vi "Find Circle.vi"(6 "Find Circle Setting":T4={"Options"={"Search  Direction"=0, "Edge Options"={"Edge Polarity"=0, "Kernel Size"=3, "Width"=3, "Minimum Edge Strength"=10.0, "Interpolation Type"=enum."Bilinear Fixed", "Data Processing Method"=enum."Average"}, "Show Search Area"=FALSE, "Show Search Lines"=FALSE, "Show Edges Found"=FALSE, "Show Result"=TRUE, "Search Area Color"=65280, "Search Lines Color"=255, "Edge Locations Color"=16776960, "Result Color"=16711680, "Overlay Group Name"=""}, "Circle Fit Options"={"Process"=enum."Get First Edge", "Step Size"=3.0, "Max Pixel Radius"=3}} {"Options"."Search  Direction" items=["Outside to Inside", "Inside to Outside"]; "Options"."Edge Options"."Edge Polarity" items=["All Edges", "Rising Edges", "Falling Edges"]; "Options"."Edge Options"."Minimum Edge Strength" format="%.2f"; "Options"."Edge Options"."Width" step=2; "Options"."Edge Options"."Kernel Size" step=2}, 8 "error in (no error)":errorcluster, 9 "Matches (pixel)":T7, 10 "ROI Descriptor":T5 {"Contours"."Type" items=["No Selection", "Point", "Line", "Rectangle", "Oval", "Polygon", "Freehand Region", "Annulus", "Unused2", "Unused3", "Broken Line", "Freehand Line", "Rotated Rectangle"]}, 11 "Image":T6) -> (0 "error out":errorcluster, 1 "Fitted Circle":T1, 2 "Found Circle?":bool, 3 "Image Out":T6)   [LabVIEW 2017]
uses:
  <vilib>/vision/Image Controls.llb/IMAQ Image.ctl
  <vilib>/vision/Measure.llb/Edge Options.ctl
  <vilib>/vision/Measure.llb/Edge Polarity.ctl
  <vilib>/vision/NI_Vision_Development_Module.lvlib
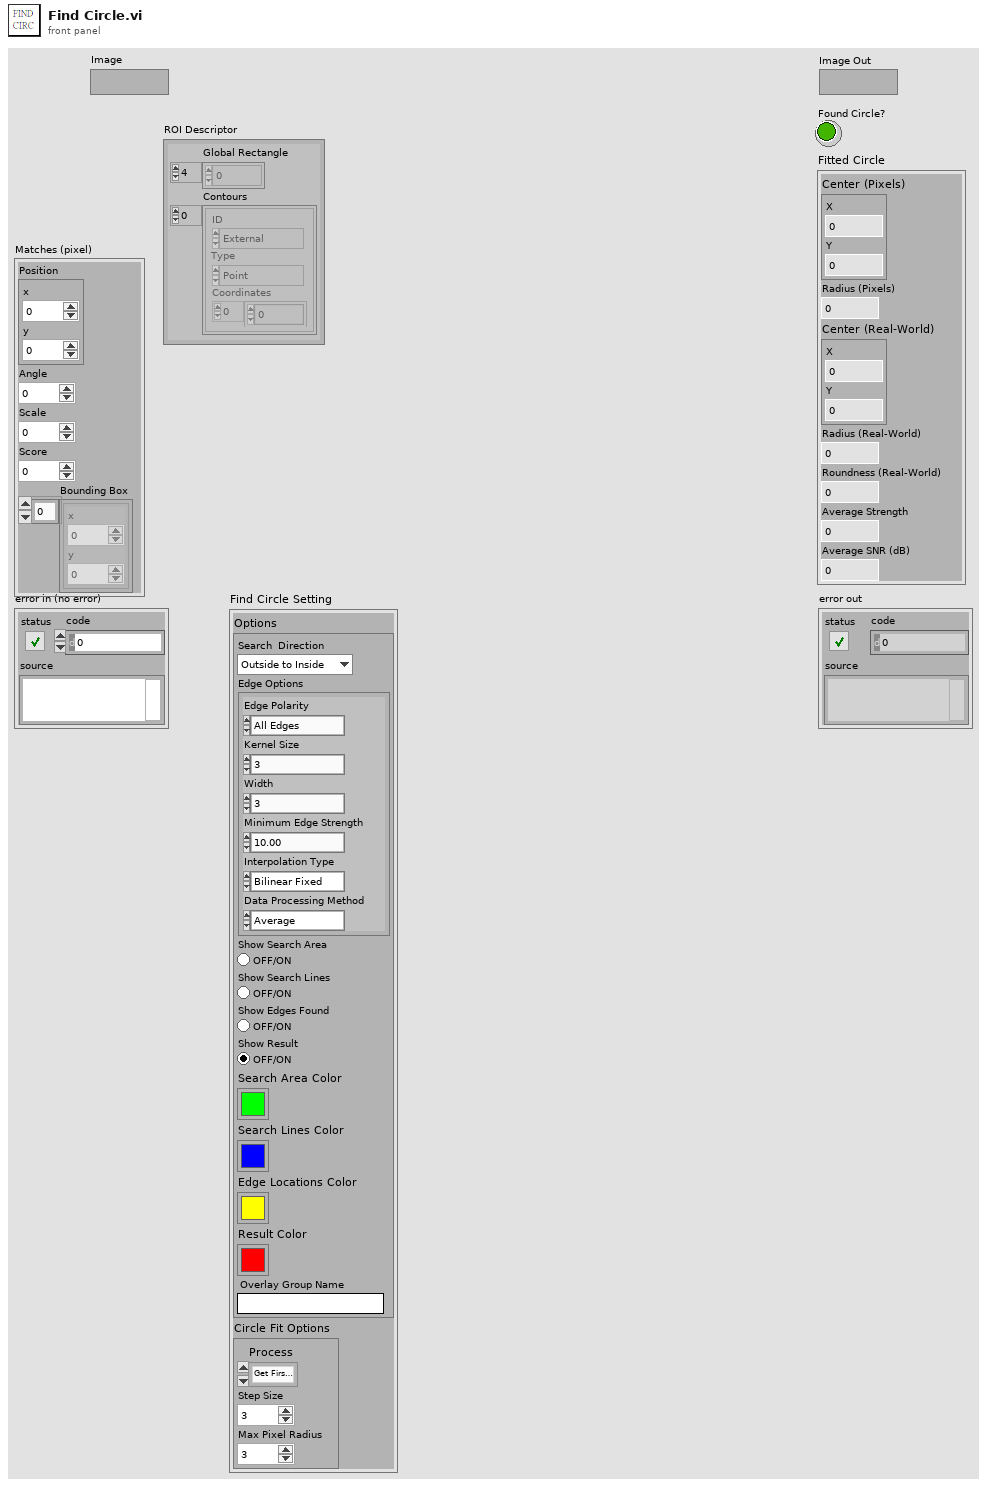
[diagram p1: front panel]
types:
  T1 = cluster{"Center (Pixels)":cluster{"X":sgl, "Y":sgl}, "Radius (Pixels)":dbl, "Center (Real-World)":cluster{"X":sgl, "Y":sgl}, "Radius (Real-World)":dbl, "Roundness (Real-World)":dbl, "Average Strength":dbl, "Average SNR (dB)":dbl}
  T2 = typedef "Edge Options.ctl" = cluster{"Edge Polarity":T3, "Kernel Size":u32, "Width":u32, "Minimum Edge Strength":sgl, "Interpolation Type":enum32{"Zero Order", "Bilinear", "Quadratic", "Cubic", "Bilinear Fixed"}, "Data Processing Method":enum32{"Average", "Median"}}
  T3 = typedef "Edge Polarity.ctl" = u32
  T4 = cluster{"Options":cluster{"Search  Direction":u32, "Edge Options":T2, "Show Search Area":bool, "Show Search Lines":bool, "Show Edges Found":bool, "Show Result":bool, "Search Area Color":u32, "Search Lines Color":u32, "Edge Locations Color":u32, "Result Color":u32, "Overlay Group Name":string}, "Circle Fit Options":cluster{"Process":enum16{"Get First Edge", "Get First + Last Edge", "Get All Edges", "Get Best Edge"}, "Step Size":dbl, "Max Pixel Radius":i32}}
  T5 = typedef "ROI Descriptor" = cluster{"Global Rectangle":i32[], "Contours":cluster{"ID":enum32{"External", "Internal"}, "Type":u32, "Coordinates":i32[]}[]}
  T6 = typedef "IMAQ Image.ctl" = refnum<image>
  T7 = cluster{"Position":cluster{"x":sgl, "y":sgl}, "Angle":sgl, "Scale":sgl, "Score":sgl, "Bounding Box":cluster{"x":sgl, "y":sgl}[]}
  T8 = enum16{"Horizontal Motion only", "Vertical Motion only", "Horizontal and Vertical Motion", "Horizontal, Vertical and Angular"}
  T9 = cluster{"Search  Direction":u32, "Edge Options":T2, "Show Search Area":bool, "Show Search Lines":bool, "Show Edges Found":bool, "Show Result":bool, "Search Area Color":u32, "Search Lines Color":u32, "Edge Locations Color":u32, "Result Color":u32, "Overlay Group Name":string}
  T10 = cluster{"Process":enum16{"Get First Edge", "Get First + Last Edge", "Get All Edges", "Get Best Edge"}, "Step Size":dbl, "Max Pixel Radius":i32}
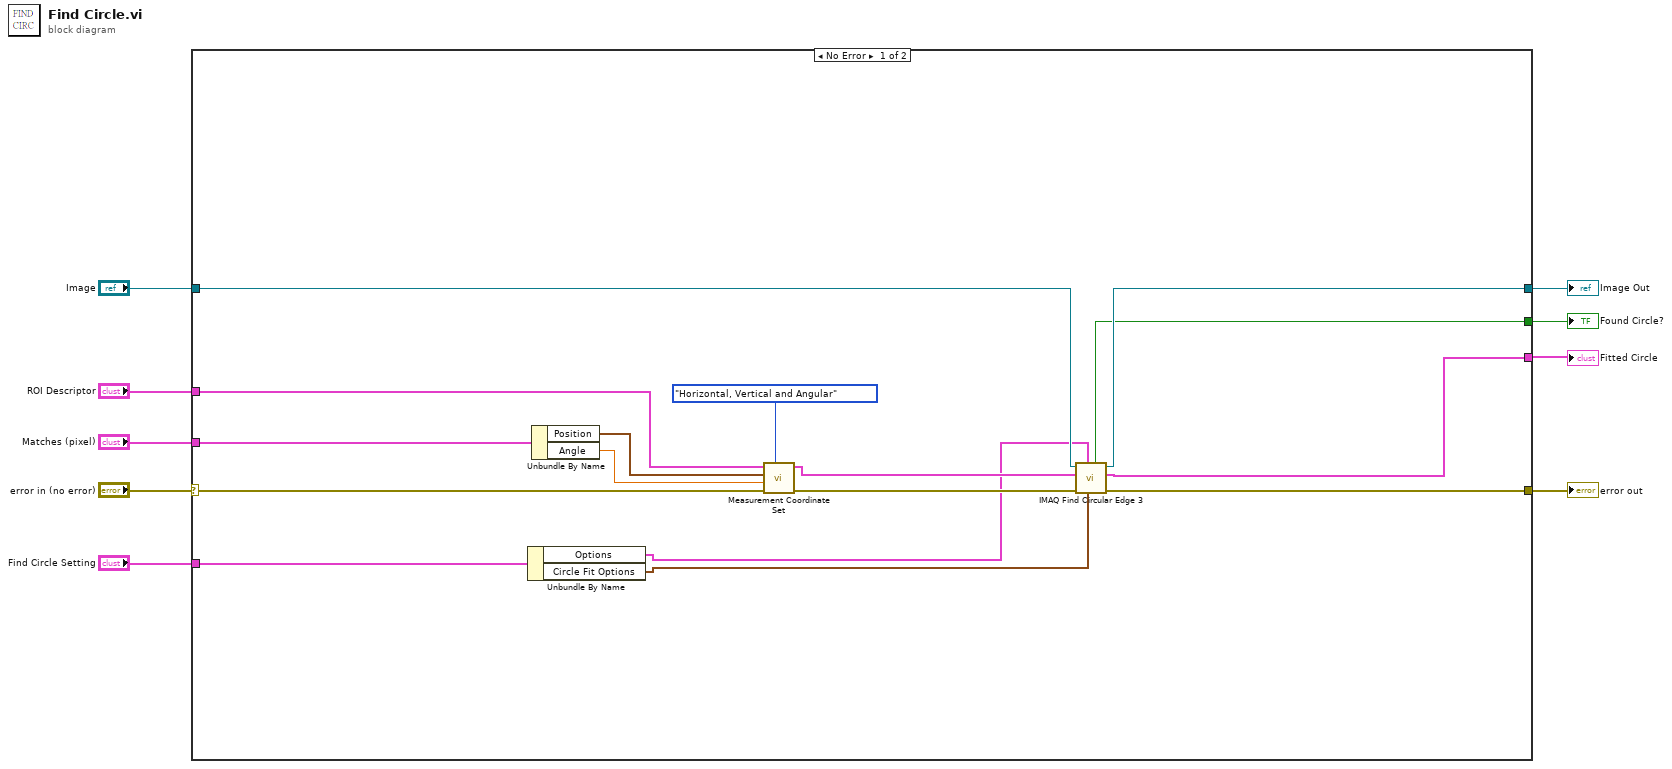
[diagram p0: block diagram]
diagram:
  n1 = case shown="No Error" "error in (no error)" {
    selector: "error in (no error)" -> [w18 w27]
    tunnel: [w23 w27] -> w8
    tunnel: "Matches (pixel)" -> [w25 _]
    tunnel: "Image" -> [w16 w26]
    tunnel: "Find Circle Setting" -> [w13 _]
    tunnel: [w22 w26] -> w5
    tunnel: [w10 _] -> w4
    tunnel: [w20 _] -> w1
    tunnel: "ROI Descriptor" -> [w15 _]
    frame No Error {
      n2 = Unbundle By Name(w13) -> ("Options"=w12:T9, "Circle Fit Options"=w11:T10)
      n3 = Unbundle By Name(w25) -> ("Position"=w24:cluster{"x":sgl, "y":sgl}, "Angle"=w21:sgl)
      n4 = call "Measurement Coordinate Set.vi"("CoordSys Type"=T8."Horizontal, Vertical and Angular", "error in (no error)"=w18, "Angle (deg)"=w21, "Origin"=w24, "ROI Descriptor"=w15) -> ("error out"=w17:errorcluster, "ROI Descriptor out"=w14:T5)  [unwired: 4 in, 1 out]
      n5 = call "IMAQ Find Circular Edge 3"("Circle Fit Options"=w11, "Options"=w12, "error in (no error)"=w17, "ROI Descriptor"=w14, "Image"=w16) -> ("error out"=w23:errorcluster, "Fitted Circle"=w20:T1, "Image Out"=w22:T6, "Circle Found"=w10:bool)  [unwired: 2 in, 1 out]
    }
    frame Error {
    }
  }
  "error out" <- w8
  "Image Out" <- w5
  "Found Circle?" <- w4
  "Fitted Circle" <- w1
